vi "Test_WriteFloat_ReadCorrectValue.vi"(8 "error in (no error)":errorcluster, 11 "TestCase in":refnum<class "TestMysqlDatabaseConfiguration.lvclass">) -> (0 "error out":errorcluster, 3 "TestCase out":refnum<class "TestMysqlDatabaseConfiguration.lvclass">)   [LabVIEW 2020, in "mysql tests.lvlib" / "TestMysqlDatabaseConfiguration.lvclass"]
uses:
  TestMysqlDatabaseConfiguration.lvclass
  TestMysqlDatabaseConfiguration.lvclass/TestMysqlDatabaseConfiguration.ctl
  <vilib>/gpm_packages/@cs/Configuration/Source/ConfigurationReference/ConfigurationReference.lvclass/ConfigurationReference.ctl
  e002e558-d5e5-459d-ba9e-71d9a5a75879.vi
  1bb3110a-552d-4b56-8dd7-594c2a54aa03.vi
  <vilib>/gpm_packages/@cs/Configuration/Source/ConfigurationReference/Explain DVR Error.vi
  e002e558-d5e5-459d-ba9e-71d9a5a75879.vi/8402ebc0-384b-46ab-989c-700e41096983.vi
  <vilib>/gpm_packages/@cs/Configuration/Source/ConfigurationReference/Read IConfiguration.vi
  <vilib>/gpm_packages/@cs/Configuration/Source/ConfigurationReference/Write IConfiguration.vi
  1bb3110a-552d-4b56-8dd7-594c2a54aa03.vi/7595dcc0-0a31-43e1-86ad-579fe37a7e85.vi
  <vilib>/gpm_packages/@cs/Configuration/Source/IConfiguration/Write SGL.vi
  <vilib>/gpm_packages/@cs/Configuration/Source/IConfiguration/Read SGL.vi
  Source/mysql-queries/mysql-queries.lvclass
  C:/Program Files/National Instruments/LabVIEW 2020/vi.lib/gpm_packages/composed-database-configuration/Source/IConfigDBQueries/IConfigurationDatabaseQueries.lvclass
  externals/mysql/Source/mysql.net/mysql.lvclass
  C:/Program Files/National Instruments/LabVIEW 2020/vi.lib/gpm_packages/composed-database-configuration/externals/database-interface/Source/IDatabase/IDatabase/IDatabase.lvclass
  Source/configuration-database.lvclass
  C:/Program Files/National Instruments/LabVIEW 2020/vi.lib/gpm_packages/@cs/Configuration/Source/IConfiguration/IConfiguration.lvclass
  <vilib>/gpm_packages/@cs/Configuration/Source/IConfiguration/IConfiguration.lvclass
  <vilib>/gpm_packages/@cs/Configuration/Source/ConfigurationReference/ConfigurationReference.lvclass
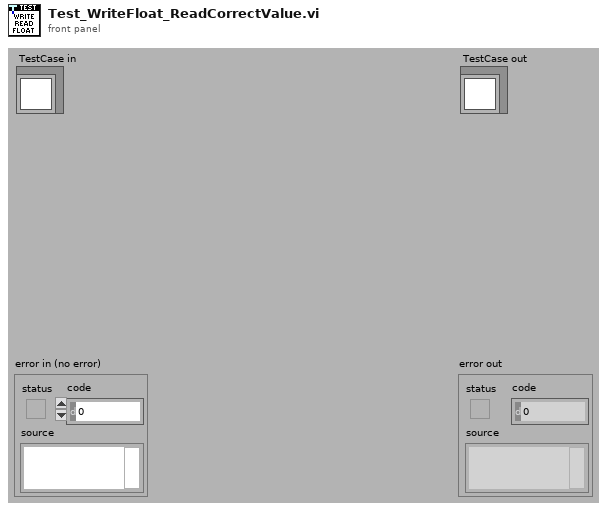
[diagram p1: front panel]
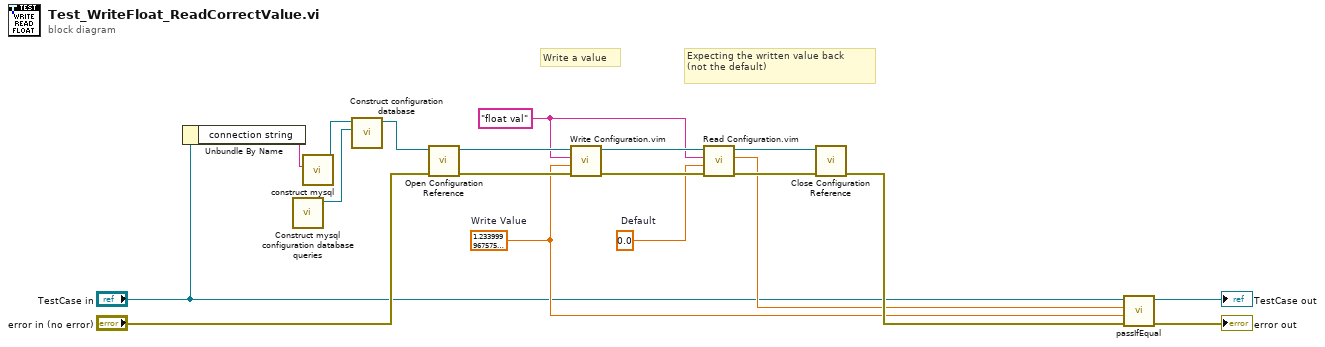
[diagram p0: block diagram]
diagram:
  w11 = sgl 0.0  # Default
  w6 = sgl 1.234  # Write Value
  w12 = "float val" ("Name")
  # "Write a value"
  # "Expecting the written value back\n(not the default)"
  n1 = Unbundle By Name("TestCase in") -> ("connection string"=w3:string)
  n2 = call "Construct mysql configuration database queries.vi"() -> ("mysql-configdb-queries out"=w1:refnum<class "mysql-queries.lvclass">)  [unwired: 10 in, 1 out]
  n3 = call "construct mysql.vi"("Connection string"=w3) -> ("mysql out"=w2:refnum<class "mysql.lvclass">)  [unwired: 9 in, 1 out]
  n4 = call "Construct configuration database.vi"("SQL logic type"=w1, "Database type in"=w2) -> ("database-configuration out"=w5:refnum<class "configuration-database.lvclass">)  [unwired: 8 in, 1 out]
  n5 = call <vilib>:"Open Configuration Reference.vi"("error in (no error)"="error in (no error)", "Configuration Type"=w5) -> ("error out"=w13:errorcluster, "Configuration Reference"=w14:refnum<data-value>)  [unwired: 8 in]
  n6 = call "Write Configuration.vim"("error in (no error)"=w13, "Value"=w6, "Name"=w12, "Configuration Reference in"=w14) -> ("error out"=w15:errorcluster, "Configuration Reference out"=w16:refnum<data-value>)  [unwired: 6 in]
  n7 = call "Read Configuration.vim"("error in (no error)"=w15, "Type (Default Value If Not Found)"=w11, "Name"=w12, "Configuration Reference in"=w16) -> ("error out"=w9:errorcluster, "Value"=w7:sgl, "Configuration Reference out"=w10:refnum<data-value>)  [unwired: 4 in, 1 out]
  n8 = call <vilib>:"Close Configuration Reference.vi"("error in (no error)"=w9, "Configuration Reference"=w10) -> ("error out"=w8:errorcluster)  [unwired: 9 in]
  n9 = call-dynamic "passIfEqual.vi"("error in (no error)"=w8, "y"=w6, "x"=w7, "TestCase in"="TestCase in") -> ("error out"=→"error out":errorcluster, "TestCase out"=→"TestCase out":refnum<class "TestMysqlDatabaseConfiguration.lvclass">)  [unwired: 6 in]
